vi "SVPO Average Dual-Channel Spectrum Measurements.vi"   [LabVIEW 2017]
doc: "Measures the frequency response of the input signals and the coherence based on the current and previous input signals. This VI returns results such as <B>Magnitude</B>, <B>Phase</B>, <B>Coherence</B>, <B>Real</B>, and <B>Imaginary</B>."
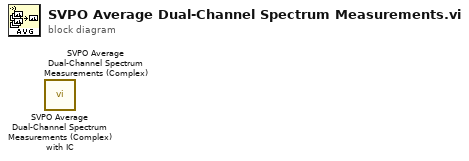
[diagram p0: block diagram]
diagram:
  n1 = call <vilib>:"SVPO Average Dual-Channel Spectrum Measurements (Complex) with IC.vi"() -> ()  [unwired: 16 in, 4 out]
  n2 = call <vilib>:"SVPO Average Dual-Channel Spectrum Measurements (Complex).vi"() -> ()  [unwired: 17 in, 3 out]
